vi "54_RC Servo Motor_default_Pulse_Width.vi"() -> ()   [LabVIEW 2018]
uses:
  <userlib>/KNR OS 4.0 LabVIEW Toolkit/Type Definition/Resource.ctl
  <userlib>/KNR OS 4.0 LabVIEW Toolkit/Type Definition/RC Servo Port.ctl
panel:
  in  "enable":bool
  in  "millisecond multiple":u32(slide)=50 scale=10.0..100.0
  in  "stop":bool
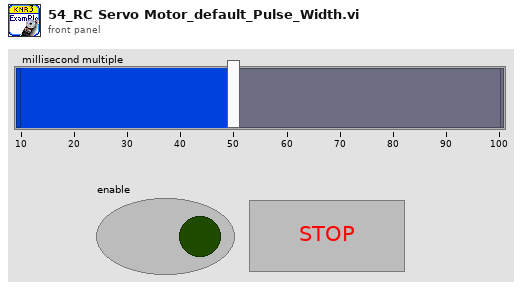
[diagram p1: front panel]
types:
  T1 = typedef "RC Servo Port.ctl" = u16
  T2 = typedef "Resource.ctl" = enum16{"KNRm_DDRC", "KNRm_DDDD", "KNRm_DDDR", "KNRm_DDDC", "KNR", "KNRm_neww"}
  T3 = typedef "KNR3 Reference.ctl" = cluster{"FPGA Session":refnum<class "FPGA Interface Base.lvclass">, "Resource":T2}
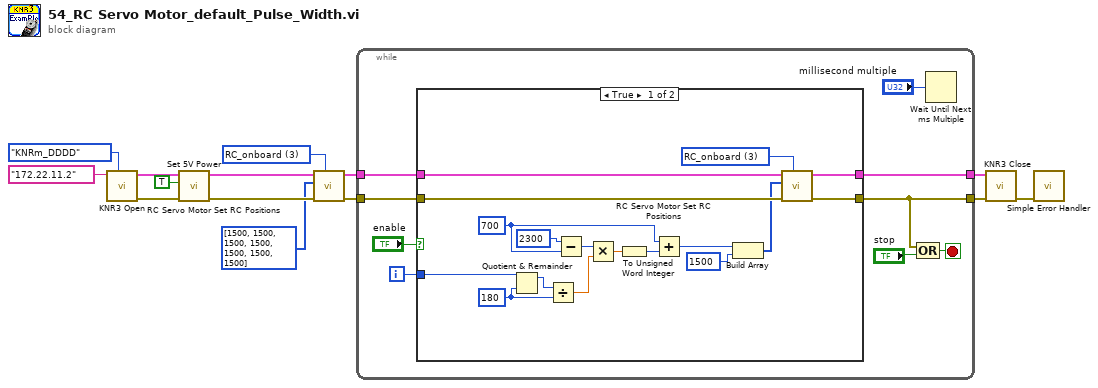
[diagram p0: block diagram]
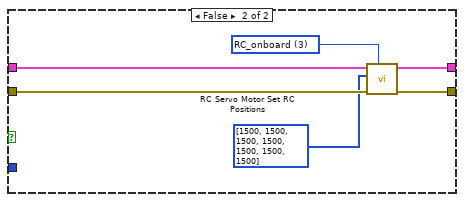
[diagram p2: hidden frame]
diagram:
  w2 = T1 3 items=["RC_onboard"=3, "RC_box"=9] ("Port (RC_onboard)")
  n1 = call <userlib>:"KNR3 Open.vi"("Resource"=Resource."KNRm_DDDD", "IP"="172.22.11.2") -> ("error out"=w11:errorcluster, "KNR out"=w13:T3)  [unwired: 8 in]
  n2 = call <userlib>:"Set 5V Power.vi"("error in (no error)"=w11, "5V Power(T)"=TRUE ("5V Power"), "KNR in"=w13) -> ("error out"=w10:errorcluster, "KNR out"=w12:T3)  [unwired: 7 in]
  n3 = call <userlib>:"RC Servo Motor Set RC Positions.vi"("Port (RC_onboard)"=w2, "RC Pulse Width (1500 uS)"=u16[] [1500, 1500, 1500, 1500, 1500, 1500, 1500], "KNR in"=w12) -> ("KNR out"=w3:T3)  [unwired: 7 in, 1 out]
  n4 = while {
    tunnel: w3 -> [w22]
    tunnel: [w21] -> w5
    tunnel: w10 -> [w20]
    tunnel: [w18] -> w4
    i -> [w15]
    stop <- w19 stop-if-true
    n5 = case shown="True" "enable" {
      tunnel: w22 -> [w39 w45]
      tunnel: [w38 w44] -> w21
      tunnel: w20 -> [w37 w43]
      tunnel: [w36 w42] -> w18
      tunnel: w15 -> [w23 _]
      frame True {
        w33 = u16 700
        w31 = u16 180 ("y")
        w35 = T1 3 items=["RC_onboard"=3, "RC_box"=9] ("RC Motor")
        n6 = Quotient & Remainder(x=w23, y=w31) -> (x-y*floor(x/y)=w32:i32)  [unwired: 1 out]
        n7 = Divide(x=w32, y=w31) -> (x/y=w29:dbl)
        n8 = Subtract(x=u16 2300, y=w33) -> (x-y=w30:u16)
        n9 = Multiply(x=w30, y=w29) -> (x*y=w28:dbl)
        n10 = To Unsigned Word Integer(number=w28) -> (unsigned 16bit integer=w27:u16)
        n11 = Add(x=w33, y=w27) -> (x+y=w25:u16)
        n12 = Build Array(w25, u16 1500) -> (w26:u16[])
        n13 = call <userlib>:"RC Servo Motor Set RC Positions.vi"("Port (RC_onboard)"=w35, "error in (no error)"=w37, "RC Pulse Width (1500 uS)"=w26, "KNR in"=w39) -> ("error out"=w36:errorcluster, "KNR out"=w38:T3)  [unwired: 6 in]
      }
      frame False {
        w41 = T1 3 items=["RC_onboard"=3, "RC_box"=9] ("RC Motor")
        n14 = call <userlib>:"RC Servo Motor Set RC Positions.vi"("Port (RC_onboard)"=w41, "error in (no error)"=w43, "RC Pulse Width (1500 uS)"=u16[] [1500, 1500, 1500, 1500, 1500, 1500, 1500], "KNR in"=w45) -> ("error out"=w42:errorcluster, "KNR out"=w44:T3)  [unwired: 6 in]
      }
    }
    n15 = Compound Arithmetic op=OR(w18, "stop") -> (w19:bool)
    n16 = Wait Until Next ms Multiple(millisecond multiple="millisecond multiple") -> ()  [unwired: 1 out]
  }
  n17 = call <userlib>:"KNR3 Close.vi"("error in (no error)"=w4, "KNR in"=w5) -> ("error out"=w9:errorcluster)  [unwired: 9 in]
  n18 = call <vilib>:"Simple Error Handler.vi"("error in (no error)"=w9) -> ()  [unwired: 4 in, 5 out]
